vi "vtktest.vi"() -> ()   [LabVIEW 2018]
uses:
  <vilib>/addons/VIRobotics/opencv_yiku/Mat/Create_Mat_8UC1_Size.vi
  <vilib>/addons/VIRobotics/opencv_yiku/Mat/Mat_8U/set2ddata.vi
  <vilib>/addons/VIRobotics/opencv_yiku/Mat/Mat_8U/Mat_8U.lvclass
  VTK-9.2.6/install/bin/vtk.dll
panel:
  out "error out":errorcluster
  out "picture":picture
  out "dims":i32[](array[numeric])
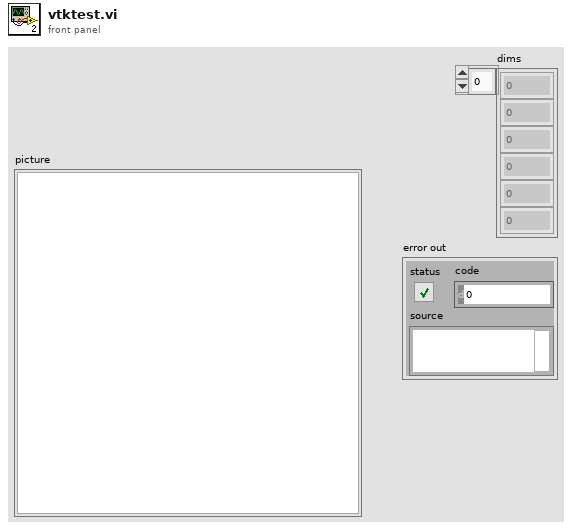
[diagram p1: front panel]
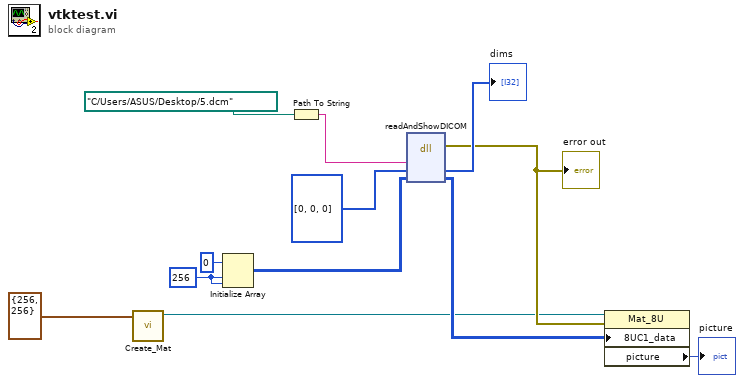
[diagram p0: block diagram]
diagram:
  w4 = 256 ("dimension size")
  n1 = call-poly <vilib>:"Create_Mat.vi"("Size"=cluster{"x":i32, "y":i32} {"x"=256, "y"=256}) -> ("Mat_8U_out"=w1:refnum<class "Mat_8U.lvclass">)  [unwired: 9 in, 1 out]
  n2 = Initialize Array(u8 0 ("element"), w4, w4) -> (w3:u8[][])
  n3 = Path To String(path=path "C:/Users/ASUS/Desktop/5.dcm") -> (string=w11:string)
  n4 = dll-call lib="C:/Users/ASUS/Desktop/VTK-9.2.6/install/bin/vtk.dll" fn="readAndShowDICOM"("filename"=w11, "dims"=i32[] [0, 0, 0], "data"=w3) -> (error out=w7:errorcluster, "dims"=→"dims":i32[], "data"=w2:u8[][])  [unwired: 5 in, 1 out]
  "error out" <- w7
  n5 = property class="Mat_8U"(reference=w1, error in=w7, "8UC1_data"=w2) -> ("picture"=→"picture":picture)  [unwired: 2 out]
